vi "Cool.vi"(0 "id":string, 1 "Set temp":string="320", 3 "error in (no error)":errorcluster) -> (7 "resulting string":string, 10 "error out":errorcluster)   [LabVIEW 2017]
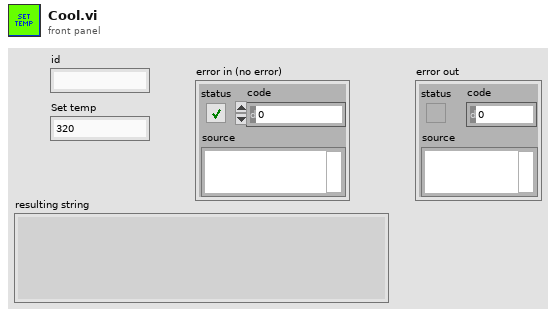
[diagram p1: front panel]
types:
  T1 = enum16{"open", "replace", "create", "open or create", "replace or create", "replace or create with confirmation"}
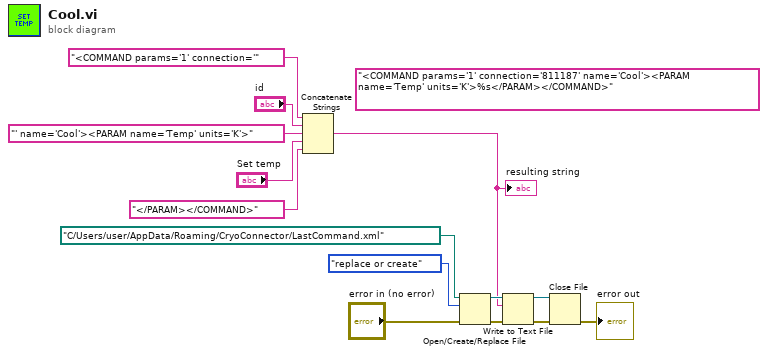
[diagram p0: block diagram]
diagram:
  (unwired) "<COMMAND params='1' connection='811187' name='Cool'><PARAM name='Temp' units='K'>%s</PARAM></COMMAND>"
  n1 = Concatenate Strings("<COMMAND params='1' connection='" ("string"), "id", "' name='Cool'><PARAM name='Temp' units='K'>" ("string"), "Set temp", "</PARAM></COMMAND>" ("string")) -> (w1:string)
  "resulting string" <- w1
  n2 = Open/Create/Replace File(file path (use dialog)=path "C:/Users/user/AppData/Roaming/CryoConnector/LastCommand.xml" ("path to XML document"), error in="error in (no error)", operation (0:open)=T1."replace or create") -> (refnum out=w10:refnum<file>, error out=w7:errorcluster)  [unwired: 3 in, 1 out]
  n3 = Write to Text File(file (use dialog)=w10, text=w1, error in=w7) -> (refnum out=w8:refnum<file>, error out=w9:errorcluster)  [unwired: 1 in, 1 out]
  n4 = Close File(refnum=w8, error in=w9) -> (error out=→"error out":errorcluster)  [unwired: 1 out]
